vi "A4988_for_stm32.vi"() -> ()   [LabVIEW 2015]
uses:
  <vilib>/Instr/_visa.llb/VISA Configure Serial Port (Instr).vi
panel:
  in  "VISA resource name":refnum<visa-resource-name>
  out "String":string
  in  "Boolean":bool
  in  "stop":bool
  out "Current position":dbl
  in  "?":u64(knob)=1 min=1 max=16 scale=1.0..16.0
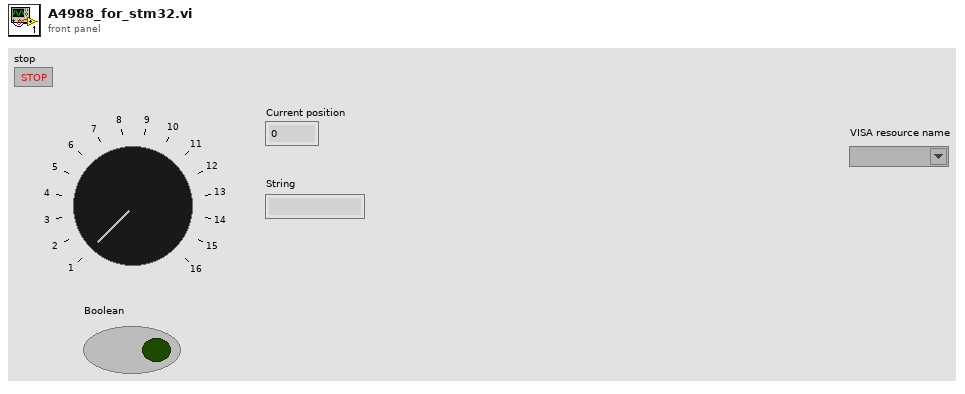
[diagram p1: front panel]
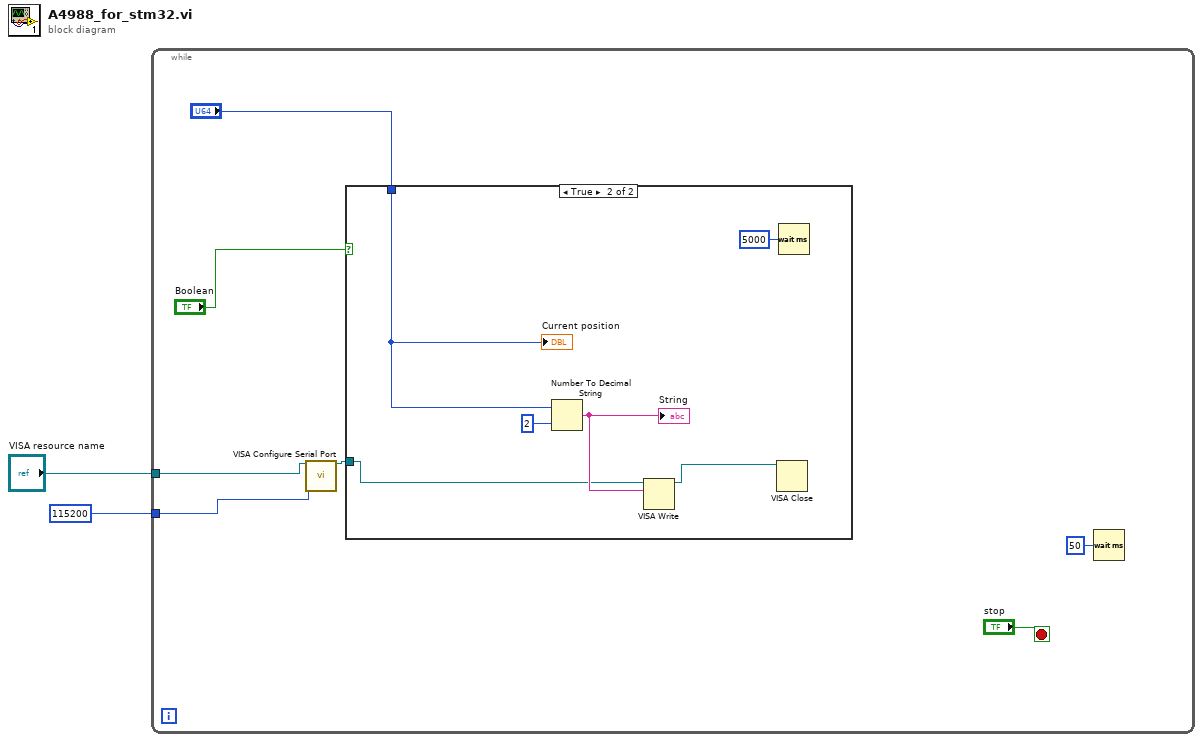
[diagram p0: block diagram]
diagram:
  n1 = while {
    tunnel: "VISA resource name" -> [w5]
    tunnel: u32 115200 ("baud rate (9600)") -> [w4]
    stop <- "stop" stop-if-true
    n2 = call-poly "VISA Configure Serial Port"("VISA resource name"=w5, "baud rate (9600)"=w4) -> ("VISA resource name out"=w6:refnum<visa-resource-name>)  [unwired: 12 in, 1 out]
    n3 = case shown="True" "Boolean" {
      tunnel: "?" -> [_ w14]
      tunnel: w6 -> [_ w11]
      frame False {
      }
      frame True {
        n4 = Number To Decimal String(number=w14, width (-)=i16 2) -> (decimal integer string=w13:string)
        "String" <- w13
        n5 = VISA Write(VISA resource name=w11, write buffer=w13) -> (VISA resource name out=w12:refnum<visa-resource-name>)  [unwired: 1 in, 2 out]
        n6 = VISA Close(VISA resource name=w12) -> ()  [unwired: 1 in, 1 out]
        n7 = Wait (ms)(milliseconds to wait=u32 5000) -> ()  [unwired: 1 out]
        "Current position" <- w14
      }
    }
    n8 = Wait (ms)(milliseconds to wait=u32 50) -> ()  [unwired: 1 out]
  }
